vi "CO TCP Packet.vi"(0 "ID":string, 5 "Version":string, 7 "utc_time":u32, 9 "PTP Sync":string="0", 11 "ue9LJ temp":u16, 12 "Flight Number":string, 13 "Data Array":string[](array[string]), 14 "In_CAL?":string="0") -> (8 "TCP Binary Packet":string)   [LabVIEW 2014]
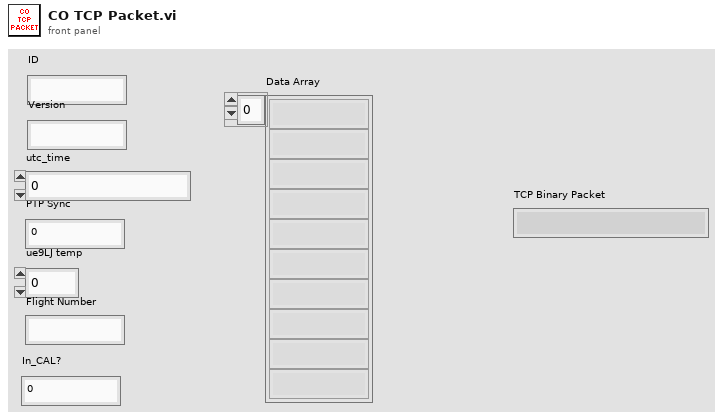
[diagram p1: front panel]
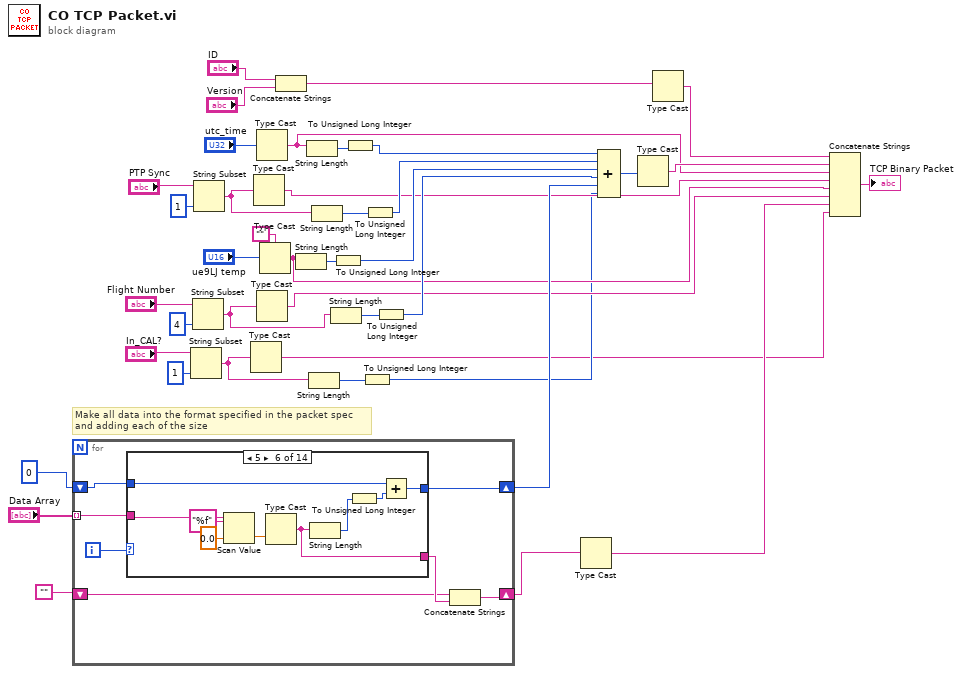
[diagram p0: block diagram]
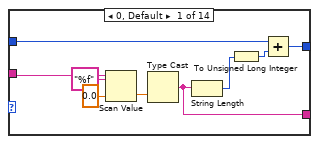
[diagram p2: hidden frame]
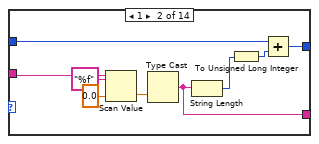
[diagram p3: hidden frame]
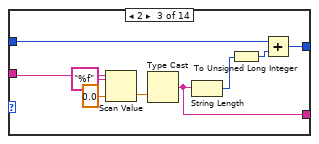
[diagram p4: hidden frame]
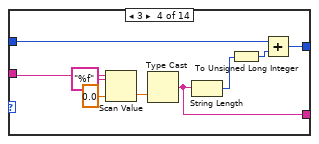
[diagram p5: hidden frame]
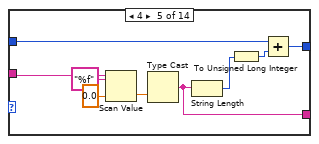
[diagram p6: hidden frame]
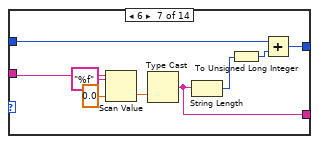
[diagram p7: hidden frame]
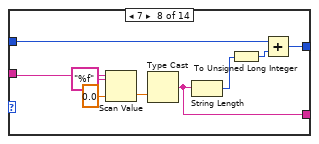
[diagram p8: hidden frame]
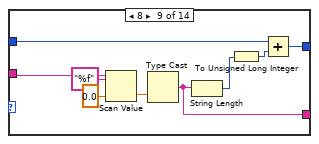
[diagram p9: hidden frame]
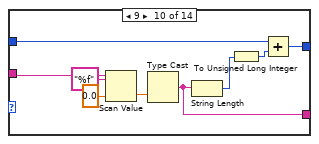
[diagram p10: hidden frame]
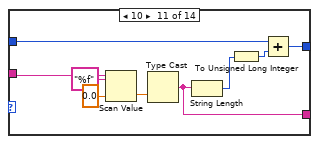
[diagram p11: hidden frame]
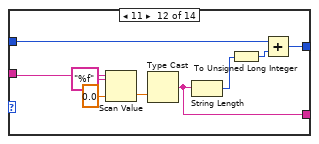
[diagram p12: hidden frame]
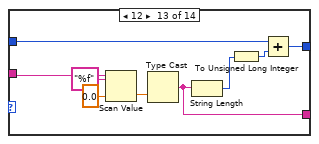
[diagram p13: hidden frame]
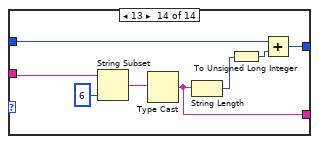
[diagram p14: hidden frame]
diagram:
  # "Make all data into the format specified in the packet spec\nand adding each of the size"
  n1 = for {
    tunnel: "Data Array" -> [w46] mode=indexing
    shift-right: [w44] -> w20
    shift-left: u32 0 -> [w45]
    shift-right: [w43] -> w7
    shift-left: "" -> [w41]
    i -> [w47]
    n2 = case shown="5" w47 {
      tunnel: w46 -> [w54 w63 w72 w81 w90 w99 w108 w117 w126 w135 w144 w153 w162 w166]
      tunnel: w45 -> [w52 w61 w70 w79 w88 w97 w106 w115 w124 w133 w142 w151 w160 w172]
      tunnel: [w49 w58 w67 w76 w85 w94 w103 w112 w121 w130 w139 w148 w157 w169] -> w44
      tunnel: [w48 w57 w66 w75 w84 w93 w102 w111 w120 w129 w138 w147 w156 w168] -> w42
      frame 0, Default {
        n3 = Scan Value(string=w54, format string="%f", default (0 dbl)=sgl 0.0 ("default (0 I32)")) -> (value=w56:sgl)  [unwired: 1 out]
        n4 = Type Cast(x=w56) -> (*(type *) &x=w48:string)  [unwired: 1 in]
        n5 = String Length(string=w48) -> (length=w51:i32)
        n6 = To Unsigned Long Integer(number=w51) -> (unsigned 32bit integer=w50:u32)
        n7 = Add(x=w52, y=w50) -> (x+y=w49:u32)
      }
      frame 1 {
        n8 = Scan Value(string=w63, format string="%f", default (0 dbl)=sgl 0.0 ("default (0 I32)")) -> (value=w65:sgl)  [unwired: 1 out]
        n9 = Type Cast(x=w65) -> (*(type *) &x=w57:string)  [unwired: 1 in]
        n10 = String Length(string=w57) -> (length=w60:i32)
        n11 = To Unsigned Long Integer(number=w60) -> (unsigned 32bit integer=w59:u32)
        n12 = Add(x=w61, y=w59) -> (x+y=w58:u32)
      }
      frame 2 {
        n13 = Scan Value(string=w72, format string="%f", default (0 dbl)=sgl 0.0 ("default (0 I32)")) -> (value=w74:sgl)  [unwired: 1 out]
        n14 = Type Cast(x=w74) -> (*(type *) &x=w66:string)  [unwired: 1 in]
        n15 = String Length(string=w66) -> (length=w69:i32)
        n16 = To Unsigned Long Integer(number=w69) -> (unsigned 32bit integer=w68:u32)
        n17 = Add(x=w70, y=w68) -> (x+y=w67:u32)
      }
      frame 3 {
        n18 = Scan Value(string=w81, format string="%f", default (0 dbl)=sgl 0.0 ("default (0 I32)")) -> (value=w83:sgl)  [unwired: 1 out]
        n19 = Type Cast(x=w83) -> (*(type *) &x=w75:string)  [unwired: 1 in]
        n20 = String Length(string=w75) -> (length=w78:i32)
        n21 = To Unsigned Long Integer(number=w78) -> (unsigned 32bit integer=w77:u32)
        n22 = Add(x=w79, y=w77) -> (x+y=w76:u32)
      }
      frame 4 {
        n23 = Scan Value(string=w90, format string="%f", default (0 dbl)=sgl 0.0 ("default (0 I32)")) -> (value=w92:sgl)  [unwired: 1 out]
        n24 = Type Cast(x=w92) -> (*(type *) &x=w84:string)  [unwired: 1 in]
        n25 = String Length(string=w84) -> (length=w87:i32)
        n26 = To Unsigned Long Integer(number=w87) -> (unsigned 32bit integer=w86:u32)
        n27 = Add(x=w88, y=w86) -> (x+y=w85:u32)
      }
      frame 5 {
        n28 = Scan Value(string=w99, format string="%f", default (0 dbl)=sgl 0.0 ("default (0 I32)")) -> (value=w101:sgl)  [unwired: 1 out]
        n29 = Type Cast(x=w101) -> (*(type *) &x=w93:string)  [unwired: 1 in]
        n30 = String Length(string=w93) -> (length=w96:i32)
        n31 = To Unsigned Long Integer(number=w96) -> (unsigned 32bit integer=w95:u32)
        n32 = Add(x=w97, y=w95) -> (x+y=w94:u32)
      }
      frame 6 {
        n33 = Scan Value(string=w108, format string="%f", default (0 dbl)=sgl 0.0 ("default (0 I32)")) -> (value=w110:sgl)  [unwired: 1 out]
        n34 = Type Cast(x=w110) -> (*(type *) &x=w102:string)  [unwired: 1 in]
        n35 = String Length(string=w102) -> (length=w105:i32)
        n36 = To Unsigned Long Integer(number=w105) -> (unsigned 32bit integer=w104:u32)
        n37 = Add(x=w106, y=w104) -> (x+y=w103:u32)
      }
      frame 7 {
        n38 = Scan Value(string=w117, format string="%f", default (0 dbl)=sgl 0.0 ("default (0 I32)")) -> (value=w119:sgl)  [unwired: 1 out]
        n39 = Type Cast(x=w119) -> (*(type *) &x=w111:string)  [unwired: 1 in]
        n40 = String Length(string=w111) -> (length=w114:i32)
        n41 = To Unsigned Long Integer(number=w114) -> (unsigned 32bit integer=w113:u32)
        n42 = Add(x=w115, y=w113) -> (x+y=w112:u32)
      }
      frame 8 {
        n43 = Scan Value(string=w126, format string="%f", default (0 dbl)=sgl 0.0 ("default (0 I32)")) -> (value=w128:sgl)  [unwired: 1 out]
        n44 = Type Cast(x=w128) -> (*(type *) &x=w120:string)  [unwired: 1 in]
        n45 = String Length(string=w120) -> (length=w123:i32)
        n46 = To Unsigned Long Integer(number=w123) -> (unsigned 32bit integer=w122:u32)
        n47 = Add(x=w124, y=w122) -> (x+y=w121:u32)
      }
      frame 9 {
        n48 = Scan Value(string=w135, format string="%f", default (0 dbl)=sgl 0.0 ("default (0 I32)")) -> (value=w137:sgl)  [unwired: 1 out]
        n49 = Type Cast(x=w137) -> (*(type *) &x=w129:string)  [unwired: 1 in]
        n50 = String Length(string=w129) -> (length=w132:i32)
        n51 = To Unsigned Long Integer(number=w132) -> (unsigned 32bit integer=w131:u32)
        n52 = Add(x=w133, y=w131) -> (x+y=w130:u32)
      }
      frame 10 {
        n53 = Scan Value(string=w144, format string="%f", default (0 dbl)=sgl 0.0 ("default (0 I32)")) -> (value=w146:sgl)  [unwired: 1 out]
        n54 = Type Cast(x=w146) -> (*(type *) &x=w138:string)  [unwired: 1 in]
        n55 = String Length(string=w138) -> (length=w141:i32)
        n56 = To Unsigned Long Integer(number=w141) -> (unsigned 32bit integer=w140:u32)
        n57 = Add(x=w142, y=w140) -> (x+y=w139:u32)
      }
      frame 11 {
        n58 = Scan Value(string=w153, format string="%f", default (0 dbl)=sgl 0.0 ("default (0 I32)")) -> (value=w155:sgl)  [unwired: 1 out]
        n59 = Type Cast(x=w155) -> (*(type *) &x=w147:string)  [unwired: 1 in]
        n60 = String Length(string=w147) -> (length=w150:i32)
        n61 = To Unsigned Long Integer(number=w150) -> (unsigned 32bit integer=w149:u32)
        n62 = Add(x=w151, y=w149) -> (x+y=w148:u32)
      }
      frame 12 {
        n63 = Scan Value(string=w162, format string="%f", default (0 dbl)=sgl 0.0 ("default (0 I32)")) -> (value=w164:sgl)  [unwired: 1 out]
        n64 = Type Cast(x=w164) -> (*(type *) &x=w156:string)  [unwired: 1 in]
        n65 = String Length(string=w156) -> (length=w159:i32)
        n66 = To Unsigned Long Integer(number=w159) -> (unsigned 32bit integer=w158:u32)
        n67 = Add(x=w160, y=w158) -> (x+y=w157:u32)
      }
      frame 13 {
        n68 = String Subset(string=w166, length (rest)=6 ("length (rest)")) -> (substring=w165:string)  [unwired: 1 in]
        n69 = Type Cast(x=w165) -> (*(type *) &x=w168:string)  [unwired: 1 in]
        n70 = String Length(string=w168) -> (length=w171:i32)
        n71 = To Unsigned Long Integer(number=w171) -> (unsigned 32bit integer=w170:u32)
        n72 = Add(x=w172, y=w170) -> (x+y=w169:u32)
      }
    }
    n73 = Concatenate Strings(w41, w42) -> (w43:string)
  }
  n74 = String Subset(string="In_CAL?", length (rest)=1 ("length (rest)")) -> (substring=w3:string)  [unwired: 1 in]
  n75 = String Subset(string="Flight Number", length (rest)=4 ("length (rest)")) -> (substring=w11:string)  [unwired: 1 in]
  n76 = String Subset(string="PTP Sync", length (rest)=1 ("length (rest)")) -> (substring=w15:string)  [unwired: 1 in]
  n77 = Type Cast(x=w3) -> (*(type *) &x=w1:string)  [unwired: 1 in]
  n78 = Type Cast(x=w15) -> (*(type *) &x=w14:string)  [unwired: 1 in]
  n79 = Type Cast(x="utc_time") -> (*(type *) &x=w16:string)  [unwired: 1 in]
  n80 = Type Cast(x=w11) -> (*(type *) &x=w12:string)  [unwired: 1 in]
  n81 = Type Cast(type="", x="ue9LJ temp") -> (*(type *) &x=w13:string)
  n82 = Concatenate Strings("ID", "Version") -> (w38:string)
  n83 = String Length(string=w13) -> (length=w29:i32)
  n84 = String Length(string=w16) -> (length=w37:i32)
  n85 = String Length(string=w3) -> (length=w5:i32)
  n86 = String Length(string=w15) -> (length=w33:i32)
  n87 = String Length(string=w11) -> (length=w25:i32)
  n88 = To Unsigned Long Integer(number=w29) -> (unsigned 32bit integer=w27:u32)
  n89 = To Unsigned Long Integer(number=w37) -> (unsigned 32bit integer=w35:u32)
  n90 = To Unsigned Long Integer(number=w5) -> (unsigned 32bit integer=w2:u32)
  n91 = To Unsigned Long Integer(number=w33) -> (unsigned 32bit integer=w31:u32)
  n92 = To Unsigned Long Integer(number=w25) -> (unsigned 32bit integer=w23:u32)
  n93 = Type Cast(x=w7) -> (*(type *) &x=w10:string)  [unwired: 1 in]
  n94 = Compound Arithmetic op=ADD(w35, w31, w27, w23, w20, w2) -> (w18:u32)
  n95 = Type Cast(x=w18) -> (*(type *) &x=w17:string)  [unwired: 1 in]
  n96 = Type Cast(x=w38) -> (*(type *) &x=w19:string)  [unwired: 1 in]
  n97 = Concatenate Strings(w19, w17, w16, w14, w13, w12, w10, w1) -> (→"TCP Binary Packet":string)
